vi "Button_Light_PS.vi"   [LabVIEW 2012]
types:
  T1 = typedef "BotSpeak_Control.ctl" = cluster{"Address":string, "Reply EOF":string, "Hardware":string, "Retries":i8, "Timeout":i32}
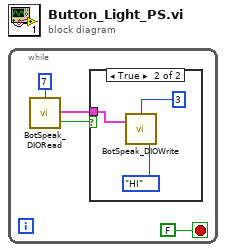
[diagram p0: block diagram]
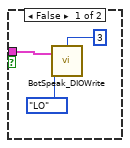
[diagram p2: hidden frame]
diagram:
  n1 = while {
    stop <- FALSE stop-if-true
    n2 = call <userlib>:"BotSpeak_DIORead.vi"("DIO Line"=u32 7) -> ("State"=w1:bool, "Bot Settings out"=w2:T1)  [unwired: 2 in]
    n3 = case shown="True" w1 {
      tunnel: w2 -> [w5 w8]
      frame False {
        n4 = call <userlib>:"BotSpeak_DIOWrite.vi"("State"=enum32{"LO", "HI"}."LO", "Bot Settings"=w5, "DIO Line"=u32 3) -> ()  [unwired: 2 out]
      }
      frame True {
        n5 = call <userlib>:"BotSpeak_DIOWrite.vi"("State"=enum32{"LO", "HI"}."HI", "Bot Settings"=w8, "DIO Line"=u32 3) -> ()  [unwired: 2 out]
      }
    }
  }
